vi "tempservice.vi"() -> ()   [LabVIEW 2009]
panel:
  in  "R45 Quad B":dbl(knob) scale=0.0..200.0
  in  "R45 quad A":dbl(knob) scale=0.0..200.0
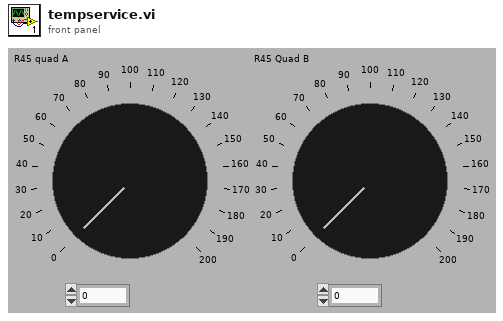
[diagram p1: front panel]
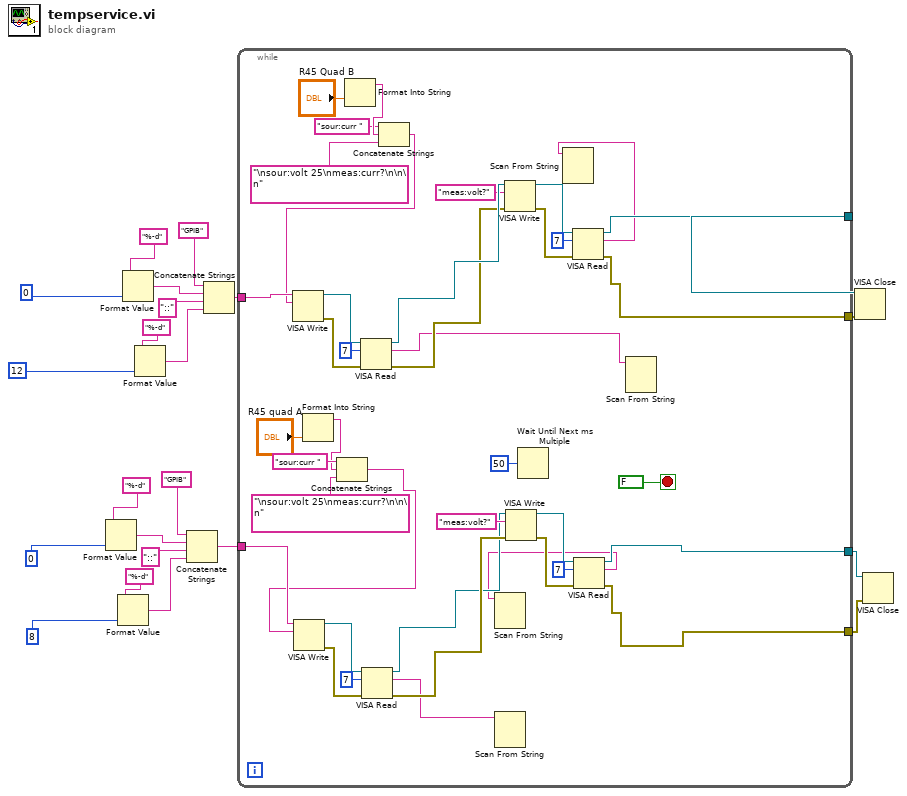
[diagram p0: block diagram]
diagram:
  n1 = Format Value(format string="%-d", value (0)=u16 0 ("Controller\nAddress(0) 2")) -> (output string=w10:string)  [unwired: 1 in]
  n2 = Format Value(format string="%-d", value (0)=u16 8 ("Device\nAddress(1) 2")) -> (output string=w5:string)  [unwired: 1 in]
  n3 = Format Value(format string="%-d", value (0)=u16 0 ("Controller\nAddress(0)")) -> (output string=w16:string)  [unwired: 1 in]
  n4 = Format Value(format string="%-d", value (0)=u16 12 ("Device\nAddress(1)")) -> (output string=w21:string)  [unwired: 1 in]
  n5 = Concatenate Strings("GPIB", w10, "::", w5) -> (w3:string)
  n6 = Concatenate Strings("GPIB", w16, "::", w21) -> (w14:string)
  n7 = while {
    tunnel: w14 -> [w62]
    tunnel: [w53] -> w13
    tunnel: [w52] -> w12
    tunnel: w3 -> [w40]
    tunnel: [w39] -> w2
    tunnel: [w38] -> w1
    stop <- FALSE stop-if-true
    n8 = Format Into String("R45 quad A") -> (resulting string=w36:string)  [unwired: 3 in, 1 out]
    n9 = Concatenate Strings("sour:curr " ("string"), w36, "\nsour:volt 25\nmeas:curr?\n\n\n" ("write buffer")) -> (w34:string)
    n10 = VISA Write(VISA resource name=w40, write buffer=w34) -> (VISA resource name out=w41:refnum<visa-resource-name>, error out=w42:errorcluster)  [unwired: 1 in, 1 out]
    n11 = Format Into String("R45 Quad B") -> (resulting string=w33:string)  [unwired: 3 in, 1 out]
    n12 = VISA Read(VISA resource name=w41, byte count=u32 7, error in (no error)=w42) -> (VISA resource name out=w47:refnum<visa-resource-name>, read buffer=w29:string, error out=w48:errorcluster)  [unwired: 1 out]
    n13 = Concatenate Strings("sour:curr " ("string"), w33, "\nsour:volt 25\nmeas:curr?\n\n\n" ("write buffer")) -> (w30:string)
    n14 = VISA Write(VISA resource name=w62, write buffer=w30) -> (VISA resource name out=w61:refnum<visa-resource-name>, error out=w60:errorcluster)  [unwired: 1 in, 1 out]
    n15 = VISA Read(VISA resource name=w61, byte count=u32 7, error in (no error)=w60) -> (VISA resource name out=w55:refnum<visa-resource-name>, read buffer=w27:string, error out=w54:errorcluster)  [unwired: 1 out]
    n16 = Scan From String(input string=w29) -> ()  [unwired: 5 in, 3 out]
    n17 = VISA Write(VISA resource name=w55, write buffer="meas:volt?", error in (no error)=w54) -> (VISA resource name out=w56:refnum<visa-resource-name>, error out=w57:errorcluster)  [unwired: 1 out]
    n18 = VISA Write(VISA resource name=w47, write buffer="meas:volt?", error in (no error)=w48) -> (VISA resource name out=w46:refnum<visa-resource-name>, error out=w45:errorcluster)  [unwired: 1 out]
    n19 = Wait Until Next ms Multiple(millisecond multiple=u32 50) -> ()  [unwired: 1 out]
    n20 = VISA Read(VISA resource name=w56, byte count=u32 7, error in (no error)=w57) -> (VISA resource name out=w53:refnum<visa-resource-name>, read buffer=w26:string, error out=w52:errorcluster)  [unwired: 1 out]
    n21 = Scan From String(input string=w26) -> ()  [unwired: 5 in, 3 out]
    n22 = VISA Read(VISA resource name=w46, byte count=u32 7, error in (no error)=w45) -> (VISA resource name out=w39:refnum<visa-resource-name>, read buffer=w28:string, error out=w38:errorcluster)  [unwired: 1 out]
    n23 = Scan From String(input string=w28) -> ()  [unwired: 5 in, 3 out]
    n24 = Scan From String(input string=w27) -> ()  [unwired: 5 in, 3 out]
  }
  n25 = VISA Close(VISA resource name=w13, error in (no error)=w12) -> ()  [unwired: 1 out]
  n26 = VISA Close(VISA resource name=w2, error in (no error)=w1) -> ()  [unwired: 1 out]
